vi "LUT_TitleScreenRed.vi"() -> (0 "Init Data Out":bool[](array[boolean]))   [LabVIEW 2018]
panel:
  # "For Initialization VI requirements and help, please read directions located on Block Diagram."
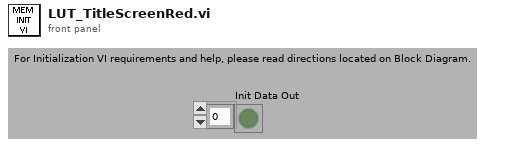
[diagram p1: front panel]
types:
  T1 = typedef "imagedata.ctl" = cluster{"image type":i32, "image depth":i32, "image":u8[], "mask":u8[], "colors":u32[], "Rectangle":cluster{"left":i16, "top":i16, "right":i16, "bottom":i16}}
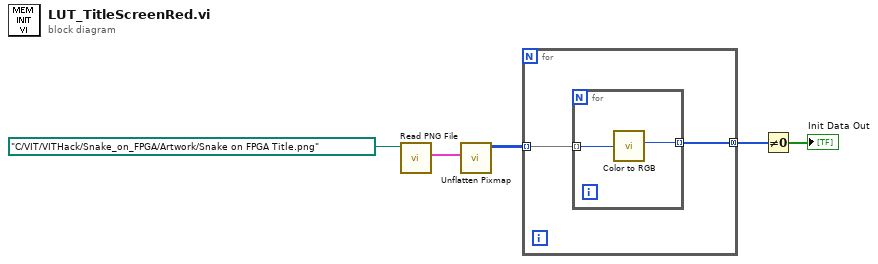
[diagram p0: block diagram]
diagram:
  n1 = call <vilib>:"Read PNG File.vi"("path to PNG file"=path "C:/VIT/VITHack/Snake_on_FPGA/Artwork/Snake on FPGA Title.png") -> ("image data"=w4:T1)  [unwired: 8 in, 2 out]
  n2 = call <vilib>:"Unflatten Pixmap.vi"("image data"=w4) -> ("24-bit pixmap"=w1:u32[][])  [unwired: 4 in, 6 out]
  n3 = for {
    tunnel: w1 -> [w7] mode=indexing
    tunnel: [w6] -> w3 mode=concatenating
    n4 = for {
      tunnel: w7 -> [w9] mode=indexing
      tunnel: [w8] -> w6 mode=indexing
      n5 = call <vilib>:"Color to RGB.vi"("Color"=w9) -> ("R"=w8:u8)  [unwired: 3 out]
    }
  }
  n6 = Not Equal To 0?(x=w3) -> (x != 0?=→"Init Data Out":bool[])
